vi "SeCrTS-DD signal names extracter.vi"(11 "input cluster":T1) -> (3 "Signal names":T2)   [LabVIEW 2022 SP3]
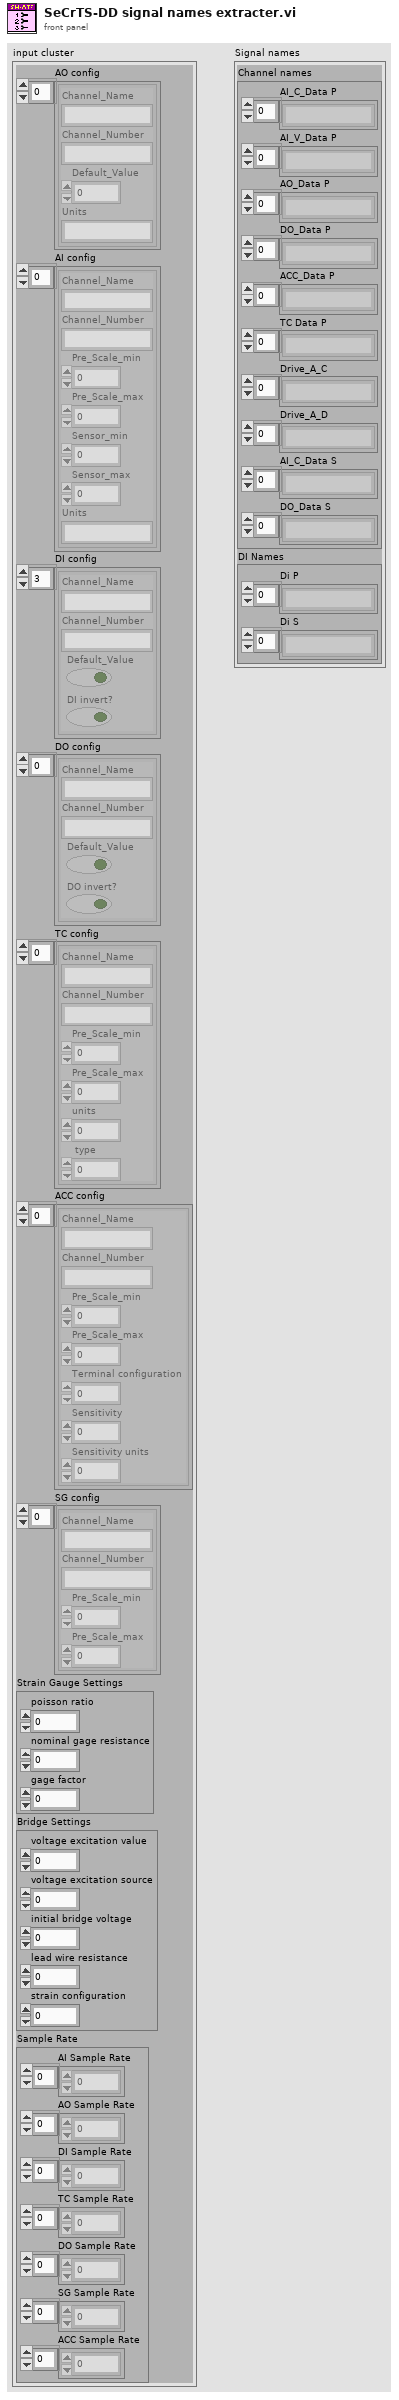
[diagram p1: front panel]
types:
  T1 = cluster{"AO config":cluster{"Channel_Name":string, "Channel_Number":string, "Default_Value":dbl, "Units":string}[], "AI config":cluster{"Channel_Name":string, "Channel_Number":string, "Pre_Scale_min":dbl, "Pre_Scale_max":dbl, "Sensor_min":dbl, "Sensor_max":dbl, "Units":string}[], "DI config":cluster{"Channel_Name":string, "Channel_Number":string, "Default_Value":bool, "DI invert?":bool}[], "DO config":cluster{"Channel_Name":string, "Channel_Number":string, "Default_Value":bool, "DO invert?":bool}[], "TC config":cluster{"Channel_Name":string, "Channel_Number":string, "Pre_Scale_min":dbl, "Pre_Scale_max":dbl, "units":i32, " type":i32}[], "ACC config":cluster{"Channel_Name":string, "Channel_Number":string, "Pre_Scale_min":dbl, "Pre_Scale_max":dbl, "Terminal configuration":i32, "Sensitivity":dbl, "Sensitivity units":i32}[], "SG config":cluster{"Channel_Name":string, "Channel_Number":string, "Pre_Scale_min":dbl, "Pre_Scale_max":dbl}[], "Strain Gauge Settings":cluster{"poisson ratio":dbl, "nominal gage resistance":dbl, "gage factor":dbl}, "Bridge Settings":cluster{"voltage excitation value":dbl, "voltage excitation source":i32, "initial bridge voltage":dbl, "lead wire resistance":dbl, "strain configuration":i32}, "Sample Rate":cluster{"AI Sample Rate":dbl[], "AO Sample Rate":dbl[], "DI Sample Rate":dbl[], "TC Sample Rate":dbl[], "DO Sample Rate":dbl[], "SG Sample Rate":dbl[], "ACC Sample Rate":dbl[]}}
  T2 = cluster{"Channel names":cluster{"AI_C_Data P":string[], "AI_V_Data P":string[], "AO_Data P":string[], "DO_Data P":string[], "ACC_Data P":string[], "TC Data P":string[], "Drive_A_C":string[], "Drive_A_D":string[], "AI_C_Data S":string[], "DO_Data S":string[]}, "DI Names":cluster{"Di P":string[], "Di S":string[]}}
  T3 = cluster{"Channel_Name":string, "Channel_Number":string, "Default_Value":dbl, "Units":string}[]
  T4 = cluster{"Channel_Name":string, "Channel_Number":string, "Pre_Scale_min":dbl, "Pre_Scale_max":dbl, "Sensor_min":dbl, "Sensor_max":dbl, "Units":string}[]
  T5 = cluster{"Channel_Name":string, "Channel_Number":string, "Default_Value":bool, "DI invert?":bool}[]
  T6 = cluster{"Channel_Name":string, "Channel_Number":string, "Default_Value":bool, "DO invert?":bool}[]
  T7 = cluster{"Channel_Name":string, "Channel_Number":string, "Pre_Scale_min":dbl, "Pre_Scale_max":dbl, "units":i32, " type":i32}[]
  T8 = cluster{"Channel_Name":string, "Channel_Number":string, "Pre_Scale_min":dbl, "Pre_Scale_max":dbl, "Terminal configuration":i32, "Sensitivity":dbl, "Sensitivity units":i32}[]
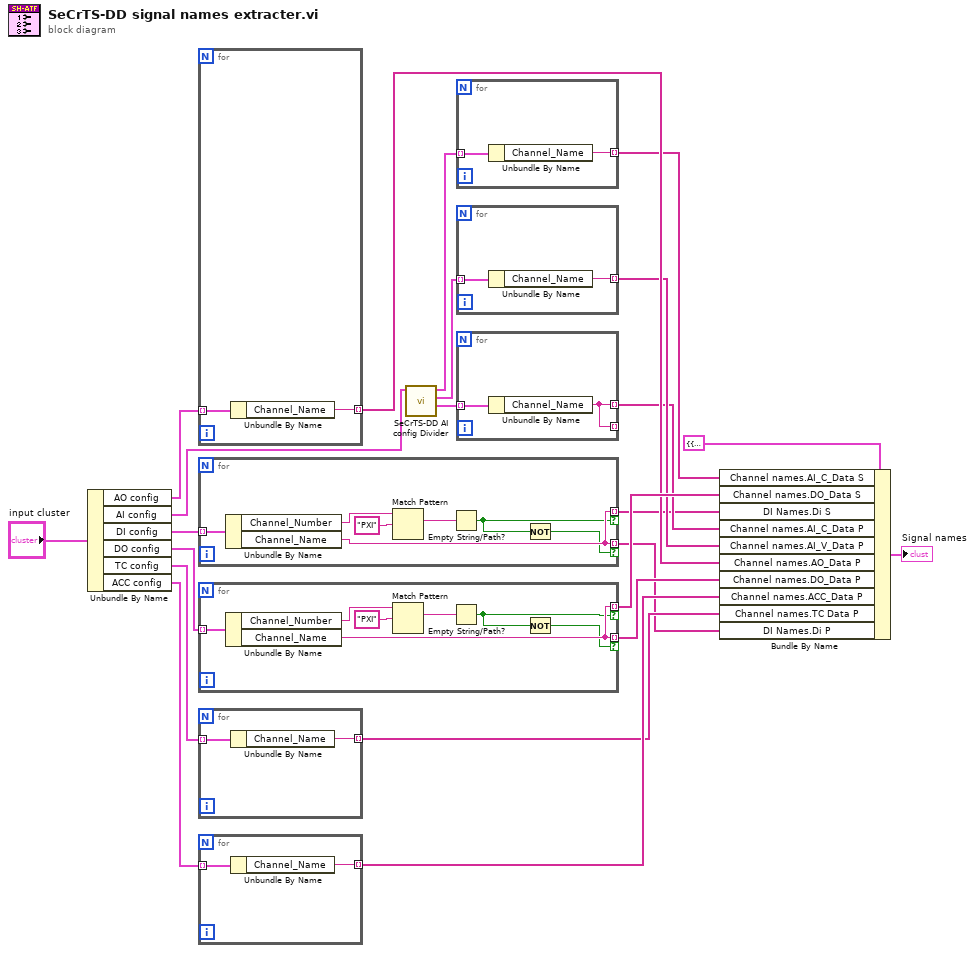
[diagram p0: block diagram]
diagram:
  n1 = Unbundle By Name("input cluster") -> ("AO config"=w15:T3, "AI config"=w20:T4, "DI config"=w16:T5, "DO config"=w17:T6, "TC config"=w18:T7, "ACC config"=w19:T8)
  n2 = for {
    tunnel: w15 -> [w24] mode=indexing
    tunnel: [w23] -> w13 mode=indexing
    n3 = Unbundle By Name(w24) -> ("Channel_Name"=w23:string)
  }
  n4 = for {
    tunnel: w16 -> [w31] mode=indexing
    tunnel: [w27] -> w2 mode=indexing if=w26
    tunnel: [w27] -> w8 mode=indexing if=w25
    n5 = Unbundle By Name(w31) -> ("Channel_Number"=w30:string, "Channel_Name"=w27:string)
    n6 = Match Pattern(string=w30, regular expression="PXI") -> (match substring=w28:string)  [unwired: 1 in, 3 out]
    n7 = Empty String/Path?(string/path=w28) -> (empty?=w26:bool)
    n8 = Not(x=w26) -> (.not. x?=w25:bool)
  }
  n9 = for {
    tunnel: w17 -> [w38] mode=indexing
    tunnel: [w37] -> w12 mode=indexing if=w33
    tunnel: [w37] -> w14 mode=indexing if=w32
    n10 = Unbundle By Name(w38) -> ("Channel_Number"=w35:string, "Channel_Name"=w37:string)
    n11 = Match Pattern(string=w35, regular expression="PXI") -> (match substring=w34:string)  [unwired: 1 in, 3 out]
    n12 = Empty String/Path?(string/path=w34) -> (empty?=w32:bool)
    n13 = Not(x=w32) -> (.not. x?=w33:bool)
  }
  n14 = for {
    tunnel: [w40] -> w10 mode=indexing
    tunnel: w18 -> [w39] mode=indexing
    n15 = Unbundle By Name(w39) -> ("Channel_Name"=w40:string)
  }
  n16 = for {
    tunnel: w19 -> [w42] mode=indexing
    tunnel: [w41] -> w11 mode=indexing
    n17 = Unbundle By Name(w42) -> ("Channel_Name"=w41:string)
  }
  n18 = call "SeCrTS-DD AI config Divider.vi"("AI config"=w20) -> ("AI C Pump"=w4:T4, "AI V Pump"=w22:T4, "AI  Storage"=w21:T4)  [unwired: 8 in]
  n19 = for {
    tunnel: w21 -> [w44] mode=indexing
    tunnel: [w43] -> w6 mode=indexing
    n20 = Unbundle By Name(w44) -> ("Channel_Name"=w43:string)
  }
  n21 = for {
    tunnel: w22 -> [w46] mode=indexing
    tunnel: [w45] -> w5 mode=indexing
    n22 = Unbundle By Name(w46) -> ("Channel_Name"=w45:string)
  }
  n23 = for {
    tunnel: w4 -> [w48] mode=indexing
    tunnel: [w47] -> _ mode=indexing
    tunnel: [w47] -> w3 mode=indexing
    n24 = Unbundle By Name(w48) -> ("Channel_Name"=w47:string)
  }
  n25 = Bundle By Name(cluster=T2 {"Channel names"={"AI_C_Data P"=[], "AI_V_Data P"=[], "AO_Data P"=[], "DO_Data P"=[], "ACC_Data P"=[], "TC Data P"=[], "Drive_A_C"=[], "Drive_A_D"=[], "AI_C_Data S"=[], "DO_Data S"=[]}, "DI Names"={"Di P"=[], "Di S"=[]}} ("Signal names"), "Channel names.AI_C_Data S"=w6, "Channel names.DO_Data S"=w14, "DI Names.Di S"=w2, "Channel names.AI_C_Data P"=w3, "Channel names.AI_V_Data P"=w5, "Channel names.AO_Data P"=w13, "Channel names.DO_Data P"=w12, "Channel names.ACC_Data P"=w11, "Channel names.TC Data P"=w10, "DI Names.Di P"=w8) -> (→"Signal names":T2)
